vi "RT_Aerodynamic_Moment_in_DLR_Navigation_Reference_System(SubVI).vi"(5 "FA":dbl[](array[numeric]), 9 "DCM":dbl[][](array[numeric]), 10 "i":i32, 11 "Data":dbl[][](array[numeric])) -> (3 "MFA (Nm)":dbl[](array[numeric]))   [LabVIEW 2017]
uses:
  <vilib>/Analysis/baseanly.llb/Real A x B.vi
  <vilib>/Analysis/Matrix/Numeric/Conversions/Array To Matrix - RA.vi
  <vilib>/Analysis/Matrix/Numeric/Conversions/Array To Matrix - RA2.vi
  <vilib>/Analysis/Matrix/Numeric/Conversions/Matrix To Array - RM.vi
  <vilib>/Analysis/NI_AALBase.lvlib
  <vilib>/Analysis/Matrix/NI_Matrix.lvlib
  <vilib>/Analysis/NI_AALPro.lvlib
panel:
  out "CoP (m)":dbl
  out "Ra":dbl[](array[numeric])
  out "ra":dbl
  out "CoG (m)":dbl
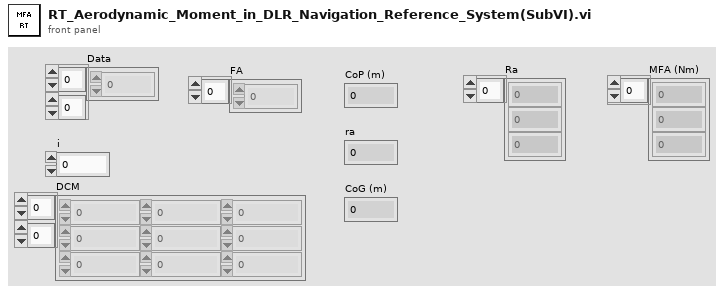
[diagram p1: front panel]
types:
  T1 = typedef "NI_Matrix.lvlib/RealMatrix.ctl" = dbl[][]
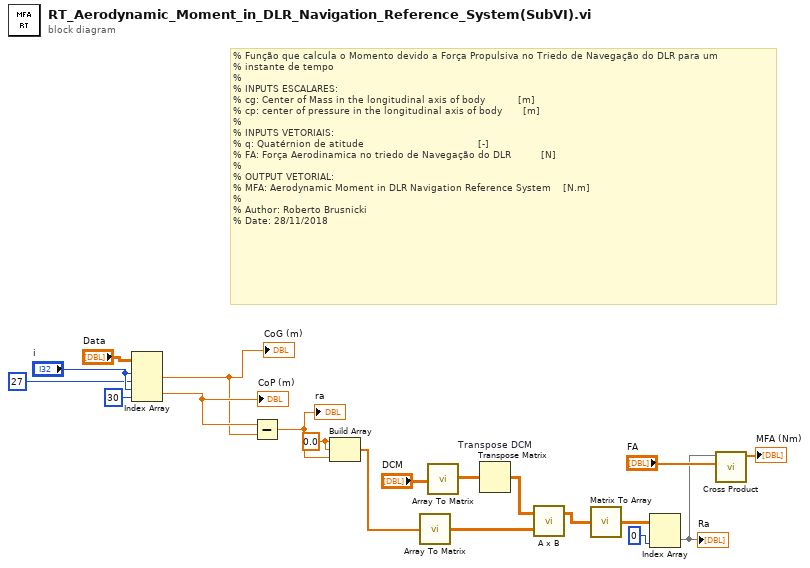
[diagram p0: block diagram]
diagram:
  w10 = 0.0 ("element")
  # "% Função que calcula o Momento devido a Força Propulsiva no Triedo de Navegação do DLR para um \n% instante de tempo\n%\n% INPUTS ESCALARES:\n% cg: Center of Mass in the longitudinal axis of body           [m]\n% cp: center of pressure in the longitudinal axis of body       [m]\n% \n% INPUTS VETORIAIS:\n% q: Quatérnion de atitude                                      [-]\n% FA: Força Aerodinamica no triedo de Navegação do DLR          [N] \t\n%\n% OUTPUT VETORIAL:\n% MFA: Aerodynamic Moment in DLR Navigation Reference System    [N.m]\n%\n% Author: Roberto Brusnicki\n% Date: 28/11/2018"
  n1 = Index Array(array="Data", index (row) #1="i", index (col) #1=27 ("disabled index (col)"), index (row) #2="i", index (col) #2=30 ("disabled index (col)")) -> (element #1=w6:dbl, element #2=w19:dbl)
  "CoG (m)" <- w6
  "CoP (m)" <- w19
  n2 = Subtract(x=w19, y=w6) -> (x-y=w11:dbl)
  "ra" <- w11
  n3 = Build Array(w10, w10, w11) -> (w9:dbl[])
  n4 = call-poly <vilib>:"Array To Matrix.vi"("Real 1D Array"=w9) -> ("Real Matrix (Column Vector)"=w12:T1)
  n5 = call-poly <vilib>:"Array To Matrix.vi"("Real 2D Array"="DCM") -> ("Real Matrix"=w8:T1)
  n6 = Transpose Matrix "Transpose DCM"(1:w8) -> (0:w7:T1)
  n7 = call-poly <vilib>:"A x B.vi"("B"=w12, "A"=w7) -> ("A x B"=w14:T1)  [unwired: 1 out]
  n8 = call-poly <vilib>:"Matrix To Array.vi"("Real Matrix"=w14) -> ("Real 2D Array"=w13:dbl[][])
  n9 = Index Array(array=w13, index (col)=0 ("index (row)")) -> (element=w4:dbl[])  [unwired: 1 in]
  "Ra" <- w4
  n10 = call <vilib>:"Cross Product.vi"("B Vector"="FA", "A Vector"=w4) -> ("Cross Product"=→"MFA (Nm)":dbl[])  [unwired: 8 in, 1 out]
